vi "SFP Self Calibrate Devices.vi"(8 "error in":errorcluster, 11 "task":refnum<k21>) -> (0 "error out":errorcluster, 2 "supported devices calibrated":bool, 3 "task":refnum<k21>)   [LabVIEW 2017]
uses:
  <resource>/objmgr/daqmx.rc
panel:
  out "documentation":string="Self calibration can take several minutes per device. You will not be able to close this dialog during self calibration. "
  in  "start":bool
  in  "done":bool
  out "Calibration Info":string[][](table)
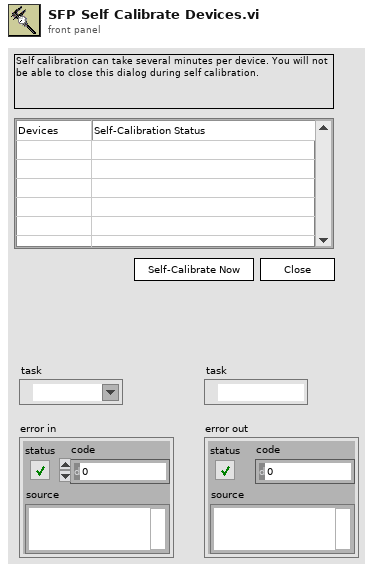
[diagram p1: front panel]
types:
  T1 = enum8{"Enabled", "Disabled", "Disabled and Grayed Out"}
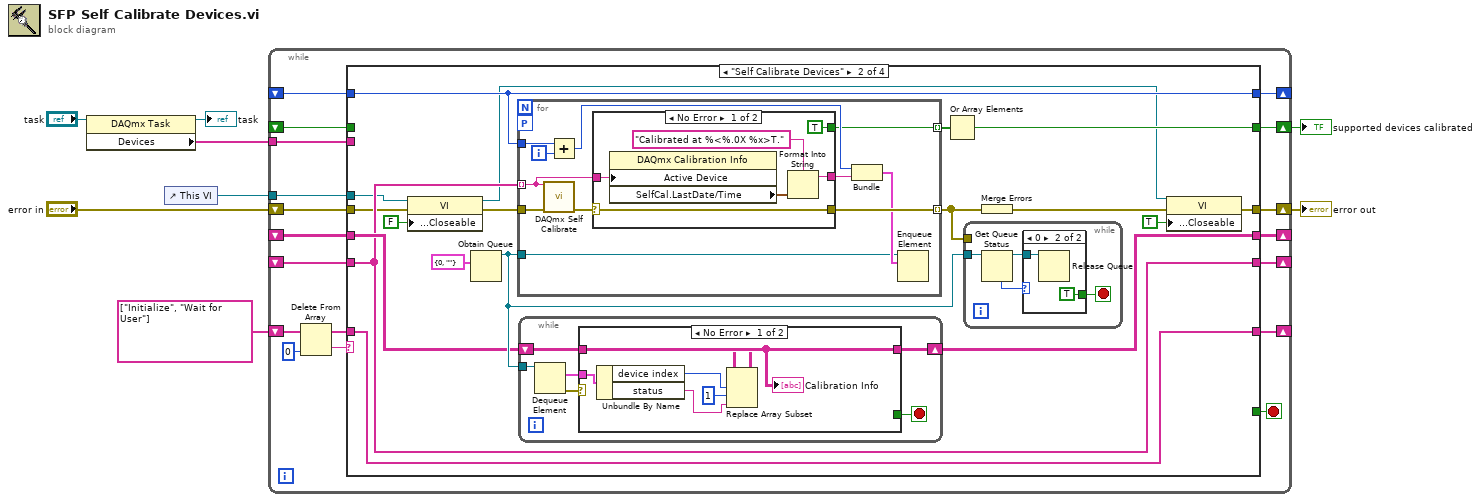
[diagram p0: block diagram]
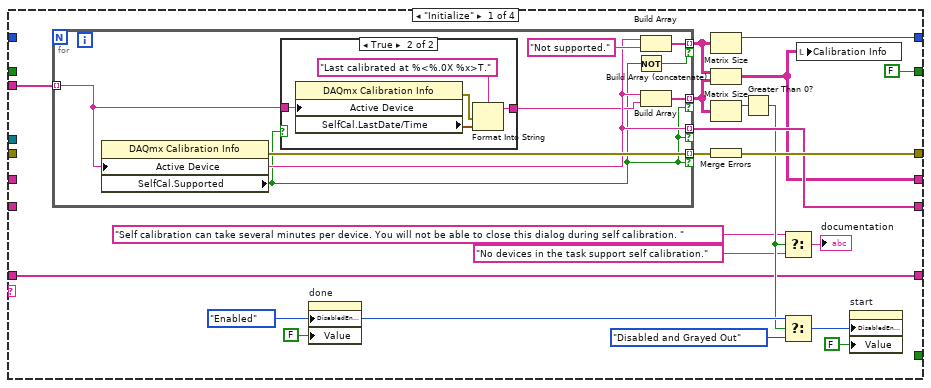
[diagram p2: hidden frame]
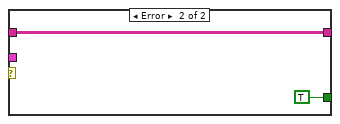
[diagram p5: hidden frame]
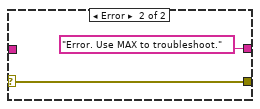
[diagram p6: hidden frame]
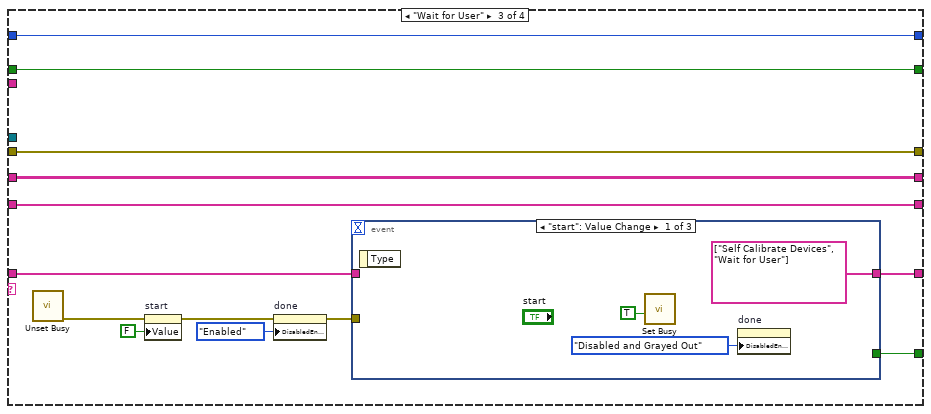
[diagram p7: hidden frame]
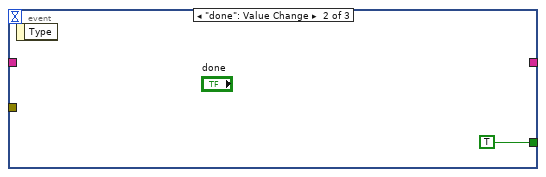
[diagram p8: hidden frame]
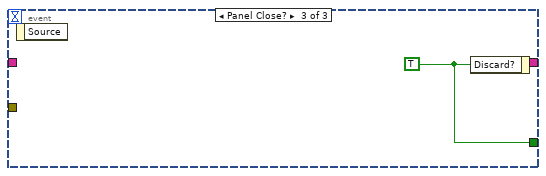
[diagram p9: hidden frame]
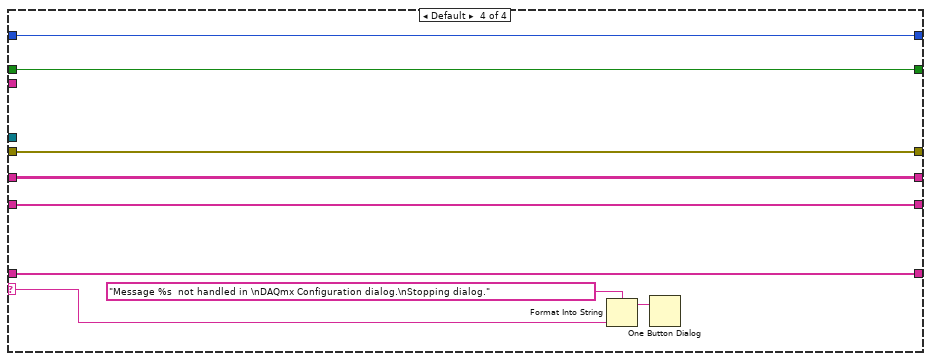
[diagram p10: hidden frame]
diagram:
  n1 = property class="DAQmx Task"(reference="task") -> (reference out=→"task":refnum<k21>, "Devices"=w3:tag[])  [unwired: 1 in, 1 out]
  n2 = control-ref of="This VI"() -> (w1:refnum<vi>)
  n3 = while {
    shift-right: [w23] -> _
    shift-left: string[] ["Initialize", "Wait for User"] -> [w25]
    shift-right: [w20] -> w6
    shift-left: "error in" -> [w21]
    shift-right: [w19] -> _
    shift-left: _ -> [w16]
    shift-right: [w18] -> _
    shift-left: _ -> [w14]
    shift-right: [w17] -> _
    shift-left: _ -> [w15]
    tunnel: w3 -> [w12]
    shift-right: [w11] -> w2
    shift-left: _ -> [w10]
    tunnel: w1 -> [w9]
    stop <- w13 stop-if-true
    n4 = Delete From Array(array=w25, index=0) -> (deleted portion=w24:string, array with subset deleted=w22:string[])  [unwired: 1 in]
    n5 = case shown="\"Self Calibrate Devices\"" w24 {
      selector: w24 -> [_ _ _ w139]
      tunnel: [w27 w60 w122 w142] -> w23
      tunnel: w22 -> [w27 w60 w123 w142]
      tunnel: w21 -> [_ w68 w125 w135]
      tunnel: [w44 w64 w125 w135] -> w20
      tunnel: [w43 w72 w128 w138] -> w19
      tunnel: [w42 w71 w126 w136] -> w18
      tunnel: [w41 w73 w127 w137] -> w17
      tunnel: w16 -> [_ w72 w128 w138]
      tunnel: w15 -> [_ w73 w127 w137]
      tunnel: w14 -> [_ w71 w126 w136]
      tunnel: [_ _ w124 _] -> w13
      tunnel: w12 -> [w29 _ _ _]
      tunnel: [FALSE w69 w116 w134] -> w11
      tunnel: w10 -> [_ _ w116 w134]
      tunnel: w9 -> [_ w66 _ _]
      frame "Initialize" {
        w39 = T1."Enabled" ("Disabled")
        n6 = for {
          tunnel: w29 -> [w49] mode=indexing
          tunnel: [w49] -> w42 mode=indexing if=w47
          tunnel: [w54] -> w45 mode=indexing if=w47
          tunnel: [w51] -> w46 mode=indexing if=w53
          tunnel: [w50] -> w40 mode=indexing if=w47
          n7 = property class="DAQmx Calibration Info"("Active Device"=w49) -> (error out=w54:errorcluster, "SelfCal.Supported"=w47:bool)  [unwired: 2 in, 1 out]
          n8 = case shown="True" w47 {
            tunnel: w49 -> [_ w59]
            tunnel: [_ w55] -> w48
            frame False {
            }
            frame True {
              n9 = property class="DAQmx Calibration Info"("Active Device"=w59) -> (error out=w57:errorcluster, "SelfCal.LastDate/Time"=w56:timestamp)  [unwired: 2 in, 1 out]
              n10 = Format Into String(format string="Last calibrated at %<%.0X %x>T.", error in=w57, w56) -> (resulting string=w55:string)  [unwired: 1 in, 1 out]
            }
          }
          n11 = Not(x=w47) -> (.not. x?=w53:bool)
          n12 = Build Array(w49, "Not supported.") -> (w51:string[])
          n13 = Build Array(w49, w48) -> (w50:string[])
        }
        n14 = property on="done" class="Bool"("DisabledEnum"=w39, "Value"=FALSE ("done")) -> ()  [unwired: 2 in, 2 out]
        n15 = Matrix Size(0:w46) -> (1:w43:i32)  [unwired: 1 out]
        n16 = Build Array (concatenate)(w46, w40) -> (w41:string[][])
        n17 = Matrix Size(0:w40) -> (1:w36:i32)  [unwired: 1 out]
        n18 = Merge Errors(w45) -> (w44:errorcluster)
        n19 = Greater Than 0?(x=w36) -> (x > 0?=w33:bool)
        n20 = Select(t="Self calibration can take several minutes per device. You will not be able to close this dialog during self calibration. " ("documentation"), s=w33, f="No devices in the task support self calibration." ("documentation")) -> (s? t:f=→"documentation":string)
        n21 = Select(t=w39, s=w33, f=T1."Disabled and Grayed Out") -> (s? t:f=w38:T1)
        n22 = local write "Calibration Info"(w41) -> ()
        n23 = property on="start" class="Bool (strict)"("DisabledEnum"=w38, "Value"=FALSE ("start")) -> ()  [unwired: 2 in, 2 out]
      }
      frame "Self Calibrate Devices" {
        n24 = property class="VI"(reference=w66, error in=w68, "Front Panel.Closeable"=FALSE ("Front Panel Window:Closeable")) -> (reference out=w63:refnum<vi>, error out=w67:errorcluster)
        n25 = Obtain Queue(element data type=cluster{"device index":i32, "status":string} {"device index"=0, "status"=""} ("cluster")) -> (queue out=w75:refnum<queue>)  [unwired: 4 in, 2 out]
        n26 = for {
          tunnel: w71 -> [w98] mode=indexing
          workers-P: _ -> [_]
          tunnel: [w105] -> w74 mode=indexing
          tunnel: w67 -> [w107]
          tunnel: w72 -> [w104]
          tunnel: w75 -> [w99]
          tunnel: [w97] -> w70 mode=indexing
          i -> [w103]
          n27 = call <vilib>:"DAQmx Self Calibrate.vi"("device in"=w98, "error in"=w107) -> ("error out"=w106:errorcluster)  [unwired: 13 in]
          n28 = Add(x=w104, y=w103) -> (x+y=w101:i32)
          n29 = case shown="No Error" w106 {
            selector: w106 -> [w110 w115]
            tunnel: w98 -> [w113 _]
            tunnel: [w110 w115] -> w105
            tunnel: [w109 "Error. Use MAX to troubleshoot."] -> w102
            tunnel: [TRUE _] -> w97
            frame No Error {
              n30 = property class="DAQmx Calibration Info"("Active Device"=w113) -> ("SelfCal.LastDate/Time"=w111:timestamp)  [unwired: 2 in, 2 out]
              n31 = Format Into String(format string="Calibrated at %<%.0X %x>T.", w111) -> (resulting string=w109:string)  [unwired: 2 in, 1 out]
            }
            frame Error {
            }
          }
          n32 = Bundle(w101, w102) -> (w100:cluster{i32, string})  [unwired: 1 in]
          n33 = Enqueue Element(queue=w99, element=w100) -> ()  [unwired: 2 in, 3 out]
        }
        n34 = while {
          tunnel: w75 -> [w88]
          shift-right: [w83] -> _
          shift-left: w73 -> [w84]
          stop <- w85 stop-if-true
          n35 = Dequeue Element(queue=w88) -> (element=w87:cluster{"device index":i32, "status":string}, error out=w86:errorcluster)  [unwired: 2 in, 2 out]
          n36 = case shown="No Error" w86 {
            tunnel: w87 -> [w93 _]
            tunnel: [_ TRUE] -> w85
            tunnel: w84 -> [w92 w95]
            tunnel: [w89 w95] -> w83
            frame No Error {
              n37 = Unbundle By Name(w93) -> ("device index"=w91:i32, "status"=w90:string)
              n38 = Replace Array Subset(array=w92, new element=w90, index (row)=w91, index (col)=1 ("disabled index (col)")) -> (w89:string[][])
              "Calibration Info" <- w89
            }
            frame Error {
            }
          }
        }
        n39 = Or Array Elements(Boolean array=w70) -> (logical OR=w69:bool)
        n40 = while {
          tunnel: w75 -> [w80]
          tunnel: w74 -> [_]
          stop <- w77 stop-if-true
          n41 = Get Queue Status(queue=w80) -> (queue out=w78:refnum<queue>, # elements in queue=w79:i32)  [unwired: 2 in, 6 out]
          n42 = case shown="0" w79 {
            tunnel: w78 -> [_ w82]
            tunnel: [_ TRUE] -> w77
            frame Default {
            }
            frame 0 {
              n43 = Release Queue(queue=w82) -> ()  [unwired: 2 in, 3 out]
            }
          }
        }
        n44 = Merge Errors(w74) -> (w65:errorcluster)
        n45 = property class="VI"(reference=w63, error in=w65, "Front Panel.Closeable"=TRUE ("Front Panel Window:Closeable")) -> (error out=w64:errorcluster)  [unwired: 1 out]
      }
      frame "Wait for User" {
        n46 = call <vilib>:"Unset Busy.vi"() -> ("error out"=w118:errorcluster)  [unwired: 11 in]
        n47 = property on="start" class="Bool (strict)"(error in=w118, "Value"=FALSE ("start")) -> (error out=w117:errorcluster)  [unwired: 1 in, 1 out]
        n48 = property on="done" class="Bool"(error in=w117, "DisabledEnum"=T1."Enabled" ("Disabled")) -> (error out=w120:errorcluster)  [unwired: 1 in, 1 out]
        n49 = event shown="[0] \"start\": Value Change" {
          selector: _ -> [_ _ _]
          dyn-events: _ -> [_ _ _]
          timeout: _ -> [_ _ _]
          tunnel: [_ TRUE w133] -> w124
          tunnel: w123 -> [_ _ _]
          tunnel: [string[] ["Self Calibrate Devices", "Wait for User"] _ _] -> w122
          tunnel: w120 -> [_ _ _]
          event "start": Value Change {
            n50 = event-data() -> ()  [unwired: 1 in, 1 out]
            n51 = call <vilib>:"Set Busy.vi"("disable click? (T)"=TRUE) -> ()  [unwired: 9 in, 2 out]
            n52 = property on="done" class="Bool"("DisabledEnum"=T1."Disabled and Grayed Out" ("Disabled")) -> ()  [unwired: 2 in, 2 out]
          }
          event "done": Value Change {
            n53 = event-data() -> ()  [unwired: 1 in, 1 out]
          }
          event Panel Close? {
            w133 = TRUE ("Discard?")
            n54 = event-data() -> ()  [unwired: 1 in, 1 out]
            n55 = event-data("Discard?"=w133) -> ()  [unwired: 1 in, 1 out]
          }
        }
      }
      frame Default {
        n56 = Format Into String(format string="Message %s  not handled in \nDAQmx Configuration dialog.\nStopping dialog.", w139) -> (resulting string=w140:string)  [unwired: 2 in, 1 out]
        n57 = One Button Dialog(message=w140) -> ()  [unwired: 1 in, 1 out]
      }
    }
  }
  "error out" <- w6
  "supported devices calibrated" <- w2
